vi "Read Serial Settings.vi"(8 "Error In":errorcluster, 11 "SerialComm in":refnum<class "SerialComm.lvclass">) -> (0 "Erorr Out":errorcluster, 2 "Serial Settings":T1={"baud rate"=9600, "data bits"=8, "parity"=enum."None", "stop bits"=10, "flow control"=0} {"flow control" items=["None"=0, "XON/XOFF"=1, "RTS/CTS"=2, "DTR/DSR"=4]; "stop bits" items=["1.0"=10, "1.5"=15, "2.0"=20]; "data bits" min=5 max=8 step=1; "baud rate" items=["75"=75, "110"=110, "134"=134, "150"=150, "300"=300, "600"=600, "1200"=1200, "1800"=1800, "2400"=2400, "4800"=4800, "7200"=7200, "9600"=9600, "14400"=14400, "19200"=19200, "28800"=28800, "38400"=38400, "56000"=56000, "57600"=57600, "115200"=115200, "128000"=128000, "230400"=230400]}, 3 "SerialComm out":refnum<class "SerialComm.lvclass">)   [LabVIEW 2017, in "SerialComm.lvclass"]
uses:
  SerialComm.lvclass
  Serial - Settings.ctl
  SerialComm.lvclass/SerialComm.ctl
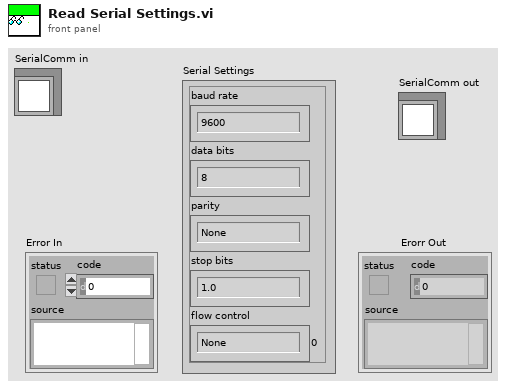
[diagram p1: front panel]
types:
  T1 = typedef "SerialComm.lvclass/Serial - Settings.ctl" = cluster{"baud rate":u32, "data bits":u16, "parity":enum16{"None", "Odd", "Even", "Mark", "Space"}, "stop bits":u16, "flow control":u16}
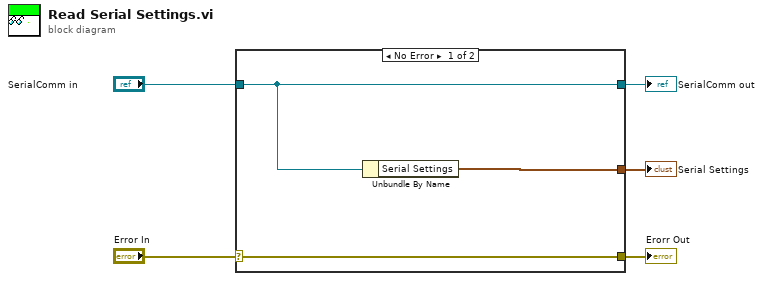
[diagram p0: block diagram]
diagram:
  n1 = case shown="No Error" "Error In" {
    selector: "Error In" -> [w8 w9]
    tunnel: [w8 w9] -> w4
    tunnel: [w7 w10] -> w2
    tunnel: "SerialComm in" -> [w7 w10]
    tunnel: [w6 _] -> w1
    frame No Error {
      n2 = Unbundle By Name(w7) -> ("Serial Settings"=w6:T1)
    }
    frame Error {
    }
  }
  "Erorr Out" <- w4
  "SerialComm out" <- w2
  "Serial Settings" <- w1
